vi "Updater.vi"() -> ()   [LabVIEW 2020]
uses:
  <vilib>/Utility/sysdir.llb/System Directory Type.ctl
  <vilib>/Utility/error.llb/Error Cluster From Error Code.vi
  <vilib>/ErrorRing/Error Ring.xnode
  <vilib>/FTP/NI_FTP.lvlib
panel:
  out "업데이터버전":string
  out "진행상황":string
  out "파일명":string
  out "진행률":string
  out "진행 막대":i32(slide) scale=-1.0..1.0
  out "업데이트?":bool
  out "에러 출력":errorcluster
  in  "에러 입력":errorcluster
  out "로컬버전":string
  out "서버버전":string
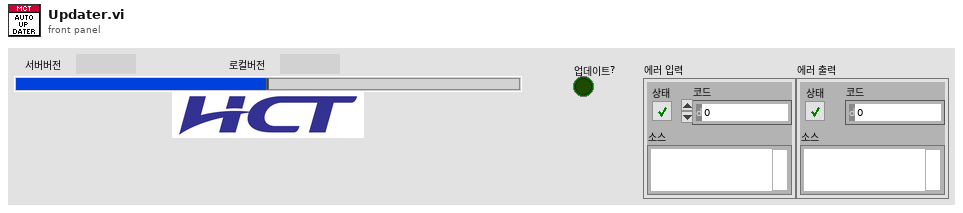
[diagram p1: front panel]
types:
  T1 = typedef "System Directory Type.ctl" = i32
  T2 = enum32{"invalid app kind", "Development System", "Run Time System", "Student Edition", "Embedded LabVIEW", "Evaluation", "Custom"}
  T3 = enum32{"Invalid", "Default", "Floating", "Floating/Auto-Hide", "Modal"}
  T4 = typedef "NI_FTP.lvlib/FTP Session.ctl" = refnum<k5>
  T5 = cluster{"로컬경로":path, "원격경로":string, "MD5 message-digest":string}[]
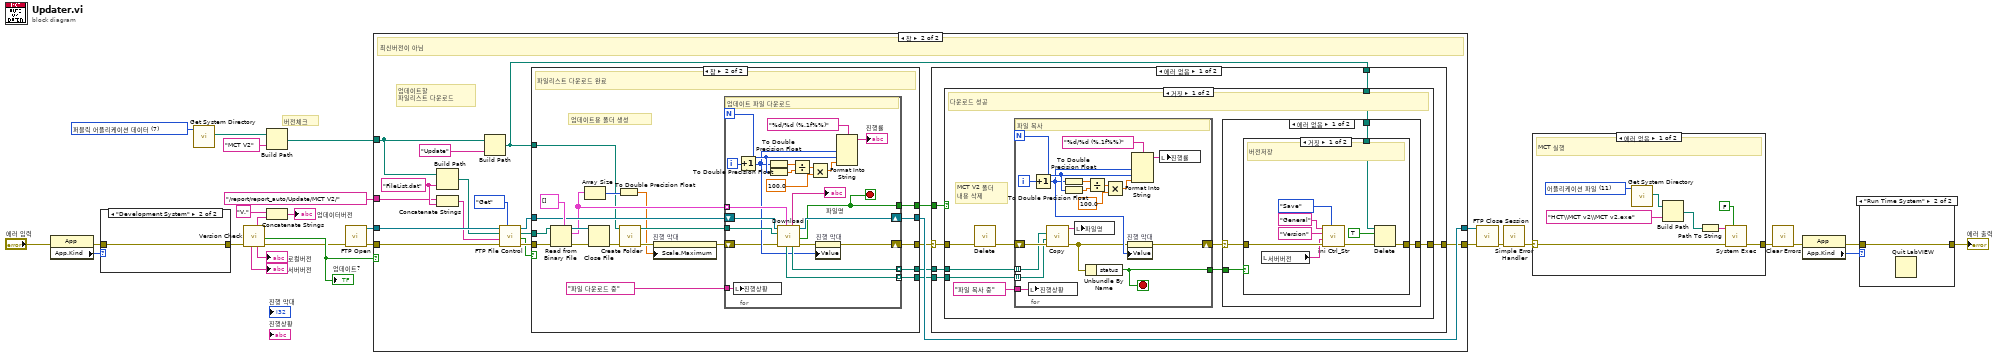
[diagram p0: block diagram]
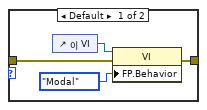
[diagram p4: hidden frame]
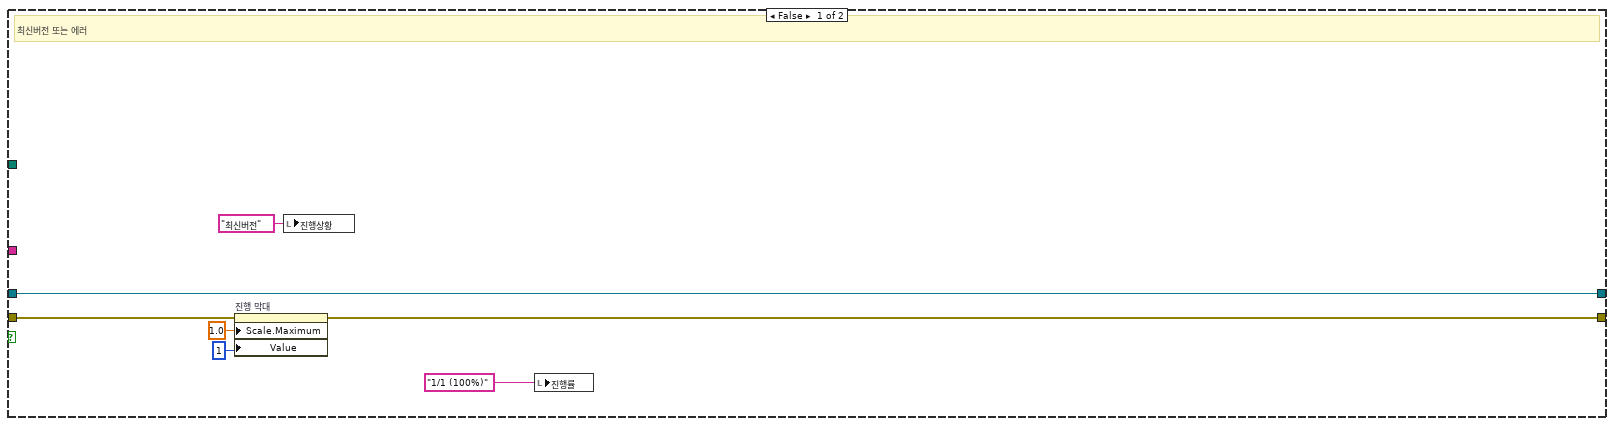
[diagram p5: hidden frame]
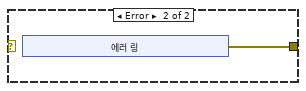
[diagram p7: hidden frame]
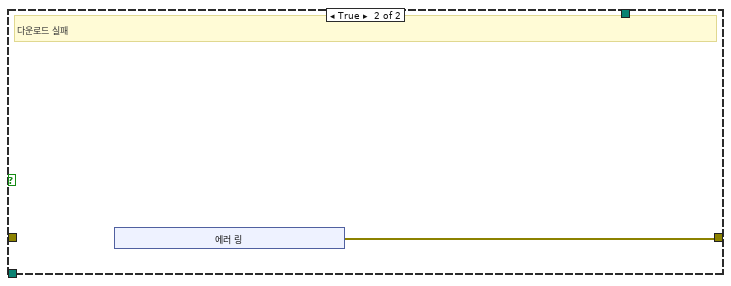
[diagram p8: hidden frame]
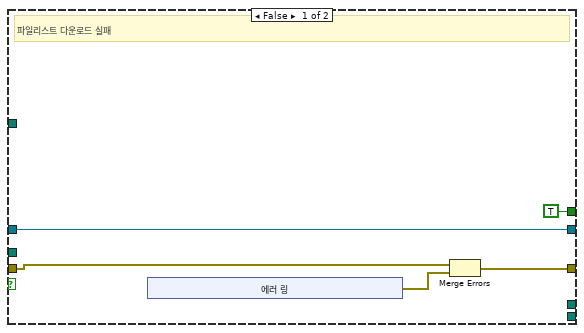
[diagram p10: hidden frame]
diagram:
  w27 = T1 7 items=["사용자 홈"=0, "사용자 데스크탑"=1, "사용자 문서"=2, "사용자 어플리케이션 데이터"=3, "사용자 환경"=4, "사용자 임시"=5, "퍼블릭 문서"=6, "퍼블릭 어플리케이션 데이터"=7, "퍼블릭 환경"=8, "퍼블릭 캐시"=13, "시스템 코어 라이브러리"=9, "시스템 설치된 라이브러리"=10, "어플리케이션 파일"=11, "부팅 볼륨 루트"=12] ("system directory type")
  # "버전체크"
  n1 = property class="App"(error in="에러 입력") -> (error out=w16:errorcluster, "App.Kind"=w17:T2)  [unwired: 1 in, 1 out]
  n2 = case shown="\"Development System\"" w17 {
    tunnel: w16 -> [w29 w32]
    tunnel: [w28 w32] -> w10
    frame Default {
      n3 = control-ref of="이 VI"() -> (w31:refnum<vi>)
      n4 = property class="VI"(reference=w31, error in=w29, "FP.Behavior"=T3."Modal" ("프런트패널 윈도우:동작")) -> (error out=w28:errorcluster)  [unwired: 1 out]
    }
    frame "Development System" {
    }
  }
  n5 = call <vilib>:"Get System Directory.vi"("system directory type"=w27) -> ("system directory"=w15:path)  [unwired: 10 in]
  n6 = call "Version Check.vi"("에러 입력"=w10) -> ("에러 출력"=w11:errorcluster, "업데이트?"=w19:bool, "MCT 로컬버전"=→"로컬버전":string, "Updater 로컬버전"=w9:string, "MCT 서버버전"=→"서버버전":string)  [unwired: 5 in, 1 out]
  "업데이트?" <- w19
  n7 = Build Path(base path=w15, name or relative path="MCT V2" ("이름 또는 상대 경로")) -> (appended path=w14:path)
  n8 = Concatenate Strings("V." ("문자열"), w9) -> (→"업데이터버전":string)
  n9 = call "FTP Open.vi"("에러 입력(에러 없음)"=w11) -> ("에러 출력"=w12:errorcluster, "TCP 네트워크 연결 출력"=w13:T4)  [unwired: 9 in]
  n10 = case shown="참" w19 {
    tunnel: w12 -> [w38 w59]
    tunnel: w13 -> [w39 w58]
    tunnel: "/report/report_auto/Update/MCT V2/" ("이름 또는 상대 경로") -> [_ w56]
    tunnel: w14 -> [_ w44]
    tunnel: [w37 w50] -> w25
    tunnel: [w39 w53] -> w24
    frame False {
      # "최신버전 또는 에러"
      n11 = property on="진행 막대" class="Slide (엄격한)"(error in=w38, "Scale.Maximum"=1.0 ("스케일.범위:최대값"), "Value"=1 ("진행 막대")) -> (error out=w37:errorcluster)  [unwired: 1 in, 1 out]
      n12 = local write "진행상황"("최신버전" ("진행상황")) -> ()
      n13 = local write "진행률"("1/1 (100%)" ("포맷 문자열")) -> ()
    }
    frame True {
      w57 = "FileList.dat" ("이름 또는 상대 경로")
      # "업데이트할\n파일리스트 다운로드"
      # "최신버전이 아님"
      n14 = Build Path(base path=w44, name or relative path=w57) -> (appended path=w40:path)
      n15 = Concatenate Strings(w56, w57) -> (w41:string)
      n16 = Build Path(base path=w44, name or relative path="Update" ("이름 또는 상대 경로")) -> (appended path=w43:path)
      n17 = call "FTP File Control.vi"("Comm"=enum16{"Get", "Put"}."Get", "에러 입력"=w59, "원격경로"=w41, "로컬경로"=w40, "TCP 네트워크 연결 입력"=w58) -> ("에러 출력"=w55:errorcluster, "파일존재?"=w52:bool, "로컬경로 out"=w51:path, "TCP 네트워크 연결 출력"=w54:T4)  [unwired: 2 in, 1 out]
      n18 = case shown="참" w52 {
        tunnel: w55 -> [w120 w149]
        tunnel: [w121 w142] -> w46
        tunnel: w54 -> [w124 w145]
        tunnel: [w124 w144] -> w53
        tunnel: [TRUE ("불리언") w136] -> w49
        tunnel: w51 -> [_ w135]
        tunnel: [_ w133] -> w48
        tunnel: [_ w132] -> w47
        tunnel: w43 -> [_ w130]
        frame False {
          # "파일리스트 다운로드 실패"
          n19 = xnode "에러 링"() -> ("에러 출력"=w122:errorcluster)
          n20 = Merge Errors(w120, w122) -> (w121:errorcluster)
        }
        frame True {
          # "업데이트용 폴더 생성"
          # "파일리스트 다운로드 완료"
          n21 = Read from Binary File(5:T5 [], 8:w149, 11:w135) -> (0:w148:errorcluster, 2:w138:T5, 3:w147:refnum<file>)  [unwired: 3 in, 1 out]
          n22 = Array Size(array=w138) -> (size(s)=w137:i32)
          n23 = Close File(refnum=w147, error in=w148) -> (error out=w141:errorcluster)  [unwired: 1 out]
          n24 = To Double Precision Float(number=w137) -> (double precision float=w134:dbl)
          n25 = call "Create Folder.vi"("에러 입력"=w141, "폴더경로"=w130) -> ("error out"=w140:errorcluster, "dup path"=w143:path)  [unwired: 8 in]
          n26 = property on="진행 막대" class="Slide (엄격한)"(error in=w140, "Scale.Maximum"=w134) -> (error out=w139:errorcluster)  [unwired: 1 in, 1 out]
          n27 = for {
            N -> [w164]
            tunnel: w138 -> [w160] mode=indexing
            shift-right: [w150] -> w142
            shift-left: w139 -> [w152]
            tunnel: w143 -> [w171]
            shift-right: [w162] -> w144
            shift-left: w145 -> [w163]
            tunnel: [w161] -> w136
            tunnel: [w156] -> w133 mode=indexing
            tunnel: [w155] -> w132 mode=indexing
            tunnel: "파일 다운로드 중" ("진행상황") -> [w154]
            i -> [w168]
            stop <- w161 stop-if-true
            # "업데이트 파일 다운로드"
            n28 = local write "진행상황"(w154) -> ()
            n29 = Increment(x=w168) -> (x+1=w153:i32)
            n30 = To Double Precision Float(number=w153) -> (double precision float=w158:dbl)
            n31 = To Double Precision Float(number=w164) -> (double precision float=w157:dbl)
            n32 = call "Download.vi"("입력 클러스터"=w160, "에러 입력(에러 없음)"=w152, "폴더명"=w171, "TCP 네트워크 연결 입력"=w163) -> ("에러 출력"=w151:errorcluster, "다운로드 에러?"=w161:bool, "TCP 네트워크 연결 출력"=w162:T4, "타겟 경로"=w156:path, "name"=→"파일명":string, "소스 경로"=w155:path)  [unwired: 2 in]
            n33 = Divide(x=w158, y=w157) -> (x/y=w167:dbl)
            n34 = Multiply(x=w167, y=100.0) -> (x*y=w165:dbl)
            n35 = property on="진행 막대" class="Slide (엄격한)"(error in=w151, "Value"=w153) -> (error out=w150:errorcluster)  [unwired: 1 in, 1 out]
            n36 = Format Into String(format string="%d/%d (%.1f%%)" ("포맷 문자열"), w153, w164, w165) -> (resulting string=→"진행률":string)  [unwired: 2 in, 1 out]
          }
        }
      }
      n37 = case shown="에러 없음" w46 {
        selector: w46 -> [w61 w119]
        tunnel: [w65 w119] -> w50
        tunnel: w49 -> [w64 _]
        tunnel: w48 -> [w63 _]
        tunnel: w47 -> [w62 _]
        tunnel: w43 -> [w60 _]
        frame No Error {
          n38 = case shown="거짓" w64 {
            tunnel: [w70 w113] -> w65
            tunnel: w61 -> [w67 _]
            tunnel: w63 -> [w74 _]
            tunnel: w62 -> [w73 _]
            tunnel: w60 -> [w68 _]
            frame False {
              # "MCT V2 폴더\n내용 삭제"
              # "다운로드 성공"
              n39 = call "Delete.vi"("에러 입력"=w67) -> ("에러 출력"=w66:errorcluster)  [unwired: 10 in]
              n40 = for {
                N -> [w105]
                tunnel: w74 -> [w111] mode=indexing
                tunnel: w73 -> [w102] mode=indexing
                shift-right: [w97] -> w71
                shift-left: w66 -> [w112]
                tunnel: "파일 복사 중" ("진행상황") -> [w98]
                tunnel: [w95] -> w69
                i -> [w100]
                stop <- w95 stop-if-true
                # "파일 복사"
                n41 = local write "진행상황"(w98) -> ()
                n42 = Increment(x=w100) -> (x+1=w99:i32)
                n43 = call "Copy.vi"("에러 입력"=w112, "소스 경로"=w102, "타겟 경로"=w111) -> ("에러 출력"=w96:errorcluster, "name"=w101:string)  [unwired: 7 in]
                n44 = To Double Precision Float(number=w99) -> (double precision float=w109:dbl)
                n45 = To Double Precision Float(number=w105) -> (double precision float=w110:dbl)
                n46 = local write "파일명"(w101) -> ()
                n47 = Unbundle By Name(w96) -> ("status"=w95:bool)
                n48 = Divide(x=w109, y=w110) -> (x/y=w106:dbl)
                n49 = Multiply(x=w106, y=100.0) -> (x*y=w108:dbl)
                n50 = property on="진행 막대" class="Slide (엄격한)"(error in=w96, "Value"=w99) -> (error out=w97:errorcluster)  [unwired: 1 in, 1 out]
                n51 = Format Into String(format string="%d/%d (%.1f%%)" ("포맷 문자열"), w99, w105, w108) -> (resulting string=w103:string)  [unwired: 2 in, 1 out]
                n52 = local write "진행률"(w103) -> ()
              }
              n53 = case shown="에러 없음" w71 {
                selector: w71 -> [w78 _]
                tunnel: [w77 w89] -> w70
                tunnel: w69 -> [w76 _]
                tunnel: w68 -> [w75 _]
                frame No Error {
                  n54 = case shown="거짓" w76 {
                    tunnel: w78 -> [w87 w88]
                    tunnel: [w79 w88] -> w77
                    tunnel: w75 -> [w81 _]
                    frame False {
                      # "버전저장"
                      n55 = local read "서버버전"() -> (w83:string)
                      n56 = call "ini Ctrl_Str.vi"("Select"=enum16{"Save", "Load"}."Save", "에러 입력"=w87, "값"=w83, "키"="Version" ("key"), "섹션"="General" ("section")) -> ("에러 출력"=w82:errorcluster)  [unwired: 4 in, 2 out]
                      n57 = Delete(path (use dialog)=w81, entire hierarchy (F)=TRUE ("전체 계층구조(거짓)"), error in=w82) -> (error out=w79:errorcluster)  [unwired: 2 in, 2 out]
                    }
                    frame True {
                    }
                  }
                }
                frame Error {
                  n58 = xnode "에러 링"() -> ("에러 출력"=w89:errorcluster)
                }
              }
            }
            frame True {
              # "다운로드 실패"
              n59 = xnode "에러 링"() -> ("에러 출력"=w113:errorcluster)
            }
          }
        }
        frame Error {
        }
      }
    }
  }
  n60 = call <vilib>:"FTP Close Session.vi"("error in (no error)"=w25, "ftp session"=w24) -> ("error out"=w23:errorcluster)  [unwired: 6 in, 3 out]
  n61 = call <vilib>:"Simple Error Handler.vi"("error in (no error)"=w23) -> ("error out"=w1:errorcluster)  [unwired: 4 in, 4 out]
  n62 = case shown="에러 없음" w1 {
    selector: w1 -> [w175 w180]
    tunnel: [w174 w180] -> w2
    frame No Error {
      w179 = T1 11 items=["사용자 홈"=0, "사용자 데스크탑"=1, "사용자 문서"=2, "사용자 어플리케이션 데이터"=3, "사용자 환경"=4, "사용자 임시"=5, "퍼블릭 문서"=6, "퍼블릭 어플리케이션 데이터"=7, "퍼블릭 환경"=8, "퍼블릭 캐시"=13, "시스템 코어 라이브러리"=9, "시스템 설치된 라이브러리"=10, "어플리케이션 파일"=11, "부팅 볼륨 루트"=12] ("system directory type")
      # "MCT 실행"
      n63 = call <vilib>:"Get System Directory.vi"("system directory type"=w179) -> ("system directory"=w178:path)  [unwired: 10 in]
      n64 = Build Path(base path=w178, name or relative path="HCT\\MCT v2\\MCT v2.exe" ("이름 또는 상대 경로")) -> (appended path=w172:path)
      n65 = Path To String(path=w172) -> (string=w173:string)
      n66 = call <vilib>:"System Exec.vi"("wait until completion? (T)"=FALSE, "error in (no error)"=w175, "command line"=w173) -> ("error out"=w174:errorcluster)  [unwired: 5 in, 3 out]
    }
    frame Error {
    }
  }
  n67 = call <vilib>:"Clear Errors.vi"("error in (no error)"=w2) -> ("error out"=w3:errorcluster)  [unwired: 5 in, 1 out]
  n68 = property class="App"(error in=w3) -> (error out=w6:errorcluster, "App.Kind"=w5:T2)  [unwired: 1 in, 1 out]
  n69 = case shown="\"Run Time System\"" w5 {
    tunnel: w6 -> [w181 w182]
    tunnel: [w181 w182] -> w4
    frame Default {
    }
    frame "Run Time System" {
      n70 = Quit LabVIEW() -> ()  [unwired: 1 in]
    }
  }
  "에러 출력" <- w4
